vi "MAC Address Fetcher1.vi"(8 "error in (no error)":errorcluster, 11 "Search all adapters?":bool=TRUE) -> (0 "error out":errorcluster, 3 "MAC Addresses":string[](array[string]))   [LabVIEW 2013]
doc: "This VI calls a Windows shell command that fetches details of the installed Network Interface Cards. It then searches for valid Physical (MAC) Addresses and populates an array. If \"All adapters\" is set to True, then the whole array will be output. otherwise, only the first element will be output, which should correspond to the primary ethernet adapter."
panel:
  out "Shell Output":string
  # "Network card MAC Address Fetcher"
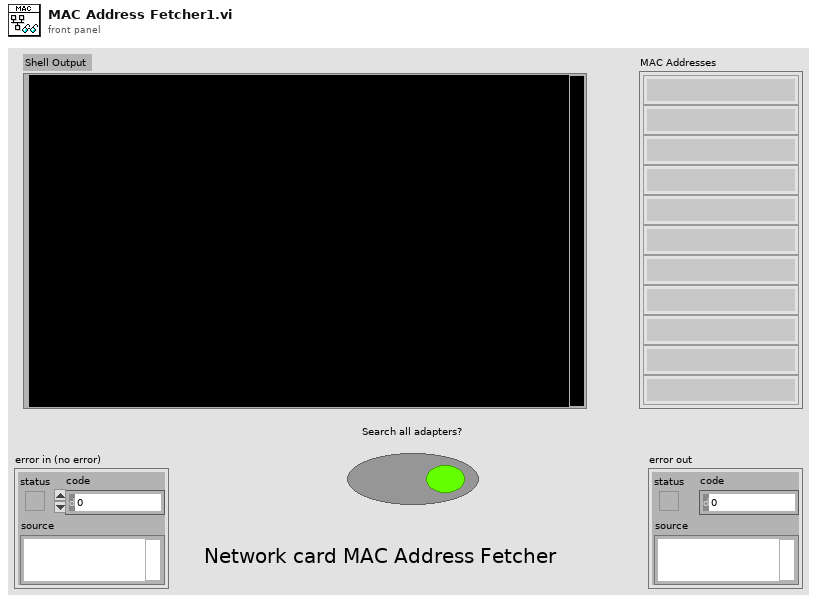
[diagram p1: front panel]
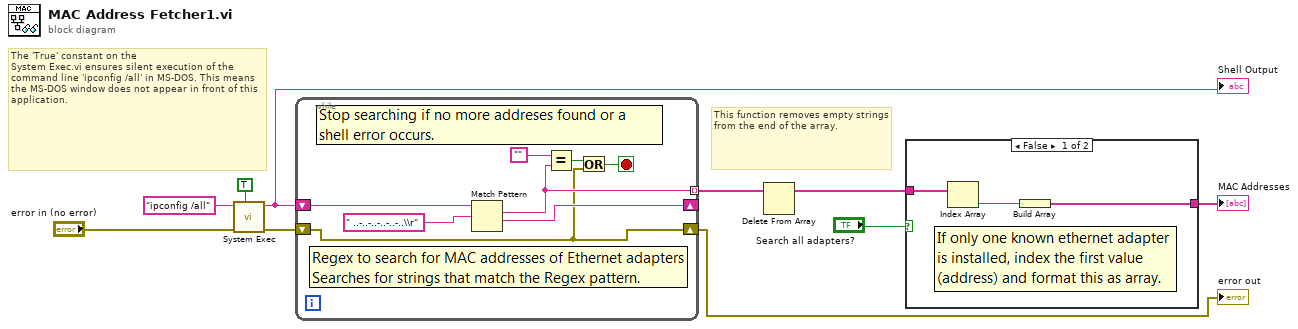
[diagram p0: block diagram]
diagram:
  # "The 'True' constant on the \nSystem Exec.vi ensures silent execution of the command line 'ipconfig /all' in MS-DOS. This means the MS-DOS window does not appear in front of this application."
  # "This function removes empty strings from the end of the array."
  n1 = call <vilib>:"System Exec.vi"("run minimized? (F)"=TRUE, "error in (no error)"="error in (no error)", "command line"="ipconfig /all") -> ("error out"=w5:errorcluster, "standard output"=w8:string)  [unwired: 5 in, 2 out]
  "Shell Output" <- w8
  n2 = while {
    shift-right: [w16] -> _
    shift-left: w8 -> [w17]
    tunnel: [w15] -> w7 mode=indexing
    shift-right: [w11] -> w4
    shift-left: w5 -> [w11]
    stop <- w12 stop-if-true
    n3 = Match Pattern(string=w17, regular expression=" ..-..-..-..-..-..\\r") -> (match substring=w15:string, after substring=w16:string)  [unwired: 1 in, 2 out]
    n4 = Equal?(x="", y=w15) -> (x = y?=w13:bool)
    n5 = Or(x=w13, y=w11) -> (x .or. y?=w12:bool)
  }
  "error out" <- w4
  n6 = Delete From Array(array=w7) -> (array with subset deleted=w2:string[])  [unwired: 2 in, 1 out]
  n7 = case shown="False" "Search all adapters?" {
    tunnel: w2 -> [w21 w22]
    tunnel: [w19 w22] -> w1
    frame False {
      n8 = Index Array(array=w21) -> (element=w20:string)  [unwired: 1 in]
      n9 = Build Array(w20) -> (w19:string[])
    }
    frame True {
      # "Otherwise, output all addresses"
    }
  }
  "MAC Addresses" <- w1
